vi "Setup_D012_R.vi"   [LabVIEW 2011]
uses:
  Modules/VisionExpressCamera.llb/VisionExpressCamera.lvclass
  Modules/PI_M126_E816Piezo.llb/PI_M126_E816Piezo.lvclass
panel:
  # "Configuration for setup in room D012, right side"
  # "Running this will open main user interface"
types:
  T1 = cluster{"VisionExpressCamera.lvclass":refnum<class "VisionExpressCamera.lvclass">, "PI_M126_E816Piezo.lvclass":refnum<class "PI_M126_E816Piezo.lvclass">}
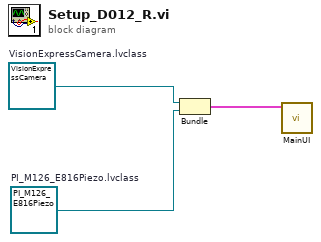
[diagram p0: block diagram]
diagram:
  w2 = refnum<class "PI_M126_E816Piezo.lvclass"> refnum  # PI_M126_E816Piezo.lvclass
  w3 = refnum<class "VisionExpressCamera.lvclass"> refnum  # VisionExpressCamera.lvclass
  n1 = Bundle("VisionExpressCamera.lvclass"=w3, "PI_M126_E816Piezo.lvclass"=w2) -> (w1:T1)  [unwired: 1 in]
  n2 = call "MainUI.vi"("Plugin List"=w1) -> ()  [unwired: 11 in]
